vi "Demo.vi"(9 "beta 2":dbl(slide)=137.76536312849163 scale=-180.0..180.0, 10 "beta 1":dbl(slide)=43.24022346368716 scale=-180.0..180.0) -> ()   [LabVIEW 2020]
uses:
  Onshape/WriteOnshapeAngle.vi
  Onshape/ReadOnshapeAngle.vi
panel:
  out "Angle2In":string="50"
  out "Angle1In":string="30"
  out "Angle1 Out":dbl
  out "Angle2 Out":dbl
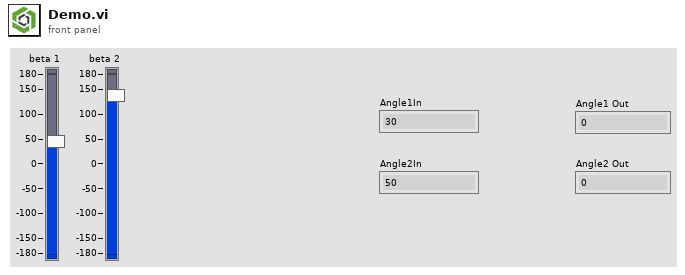
[diagram p1: front panel]
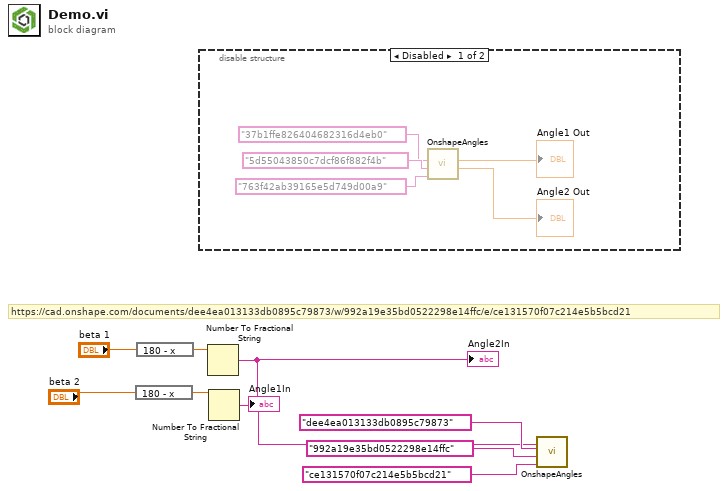
[diagram p0: block diagram]
diagram:
  # "https://cad.onshape.com/documents/dee4ea013133db0895c79873/w/992a19e35bd0522298e14ffc/e/ce131570f07c214e5b5bcd21"
  n1 = expression code="180 - x"("beta 2") -> (w6:dbl)
  n2 = expression code="180 - x"("beta 1") -> (w4:dbl)
  n3 = disable-structure shown="Disabled" {
    frame Disabled {
      n4 = call-poly "OnshapeAngles.vi"("eid"="763f42ab39165e5d749d00a9", "wid"="5d55043850c7dcf86f882f4b", "did"="37b1ffe826404682316d4eb0") -> ("Angle2Out"=→"Angle2 Out":dbl, "Angle1Out"=→"Angle1 Out":dbl)  [unwired: 6 in, 1 out]
    }
    frame Enabled {
    }
  }
  n5 = Number To Fractional String(number=w4) -> (F-format string=w3:string)  [unwired: 3 in]
  "Angle2In" <- w3
  n6 = Number To Fractional String(number=w6) -> (F-format string=w5:string)  [unwired: 3 in]
  "Angle1In" <- w5
  n7 = call-poly "OnshapeAngles.vi"("Angle2In"=w3, "Angle1In"=w5, "eid"="ce131570f07c214e5b5bcd21", "wid"="992a19e35bd0522298e14ffc", "did"="dee4ea013133db0895c79873") -> ()  [unwired: 6 in, 1 out]
